vi "HOL_Trajectory_SampleReverseTEST_CONSTORIENT.vi"(9 "Time":dbl, 11 "InputTRAJECTORY":T5 {"States"."POSE"."ROTATION"."SIN" format="%13.4f"; "States"."POSE"."ROTATION"."COS" format="%13.4f"; "States"."POSE"."ROTATION"."VALUE" format="%13.4f"; "States"."POSE"."TRANSLATION"."Y" format="%14.3f"; "States"."POSE"."TRANSLATION"."X" format="%14.3f"; "TotalTImeSecs" format="%20.3f"}) -> (3 "OutputTRAJ_STATE":T1={"TimeSeconds"=0.0, "Velocity"=0.0, "Acceleration"=0.0, "POSE"={"TRANSLATION"={"X"=0.0, "Y"=0.0}, "ROTATION"={"VALUE"=0.0, "COS"=1.0, "SIN"=0.0}}, "Curvature"=0.0} {"POSE"."ROTATION"."SIN" format="%13.4f"; "POSE"."ROTATION"."COS" format="%13.4f"; "POSE"."ROTATION"."VALUE" format="%13.4f"; "POSE"."TRANSLATION"."Y" format="%14.3f"; "POSE"."TRANSLATION"."X" format="%14.3f"})   [LabVIEW 2019]
doc: "Sample the trajectory at a point in time. The trajectory is sampled in reverse such that the ending time becomes 0 and the beginning time is the maximum time. The selected trajectory state is then transformed to be relative to end of the trajectory.\n\nThis routine does not exist in WPILIB\n \nParameters:\n - InputTrajectory - The Trajectory data structure\n - time - The point in time since the beginning of the trajectory to sample. (seconds)\n\nReturns:\n - OutputTrajState - The state at that point in time."
uses:
  <vilib>/Rock Robotics/WPI/ThirdParty/JAS_Junk/TrajLib/TRAJECTORY.ctl
  <vilib>/Rock Robotics/WPI/ThirdParty/JAS_Junk/TrajLib/TRAJ_STATE.ctl
  <vilib>/Rock Robotics/WPI/ThirdParty/JAS_Junk/TrajLib/POSE2D.ctl
  <vilib>/Rock Robotics/WPI/ThirdParty/JAS_Junk/TrajLib/TRANSLATION2D.ctl
  <vilib>/Rock Robotics/WPI/ThirdParty/JAS_Junk/TrajLib/ROTATION2D.ctl
  <vilib>/Rock Robotics/WPI/ThirdParty/JAS_Junk/TrajLib/Translation_Create.vi
  <vilib>/Rock Robotics/WPI/ThirdParty/JAS_Junk/TrajLib/Trajectory_Library.lvlib
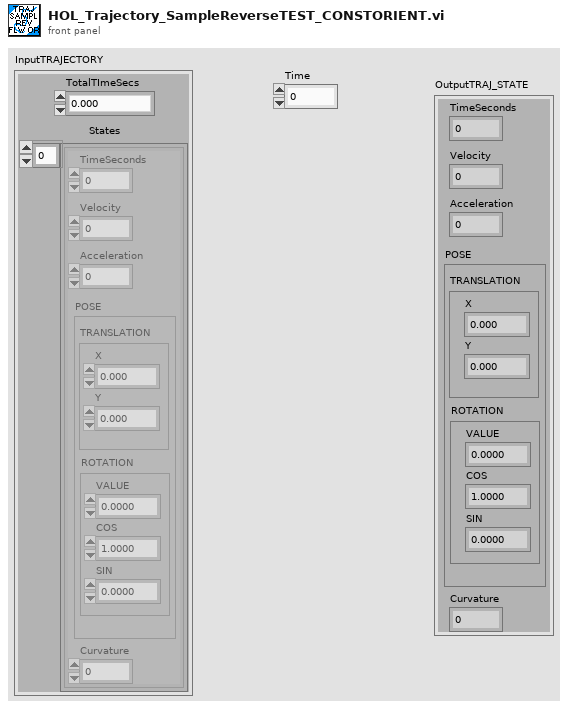
[diagram p1: front panel]
types:
  T1 = typedef "Trajectory_Library.lvlib/TRAJ_STATE.ctl" = cluster{"TimeSeconds":dbl, "Velocity":dbl, "Acceleration":dbl, "POSE":T2, "Curvature":dbl}
  T2 = typedef "Trajectory_Library.lvlib/POSE2D.ctl" = cluster{"TRANSLATION":T3, "ROTATION":T4}
  T3 = typedef "Trajectory_Library.lvlib/TRANSLATION2D.ctl" = cluster{"X":dbl, "Y":dbl}
  T4 = typedef "Trajectory_Library.lvlib/ROTATION2D.ctl" = cluster{"VALUE":dbl, "COS":dbl, "SIN":dbl}
  T5 = typedef "Trajectory_Library.lvlib/TRAJECTORY.ctl" = cluster{"TotalTImeSecs":dbl, "States":T1[]}
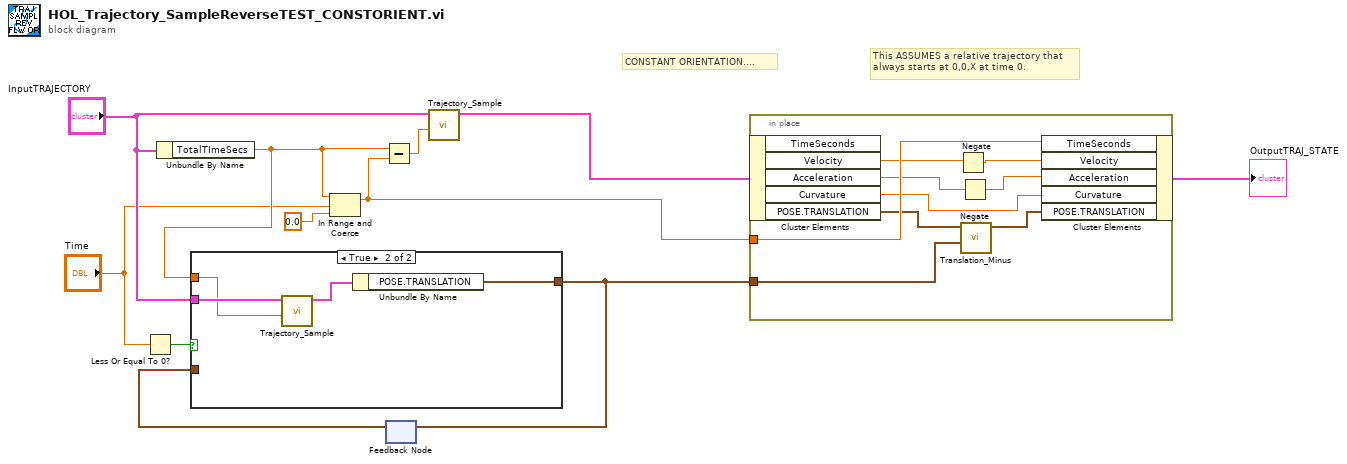
[diagram p0: block diagram]
diagram:
  # "This ASSUMES a relative trajectory that \nalways starts at 0,0,X at time 0."
  # "CONSTANT ORIENTATION...."
  n1 = Less Or Equal To 0?(x="Time") -> (x <= 0?=w11:bool)
  n2 = Unbundle By Name("InputTRAJECTORY") -> ("TotalTImeSecs"=w4:dbl)
  n3 = In Range and Coerce(upper limit=w4, x="Time", lower limit=0.0) -> (coerced(x)=w2:dbl)  [unwired: 1 out]
  n4 = Subtract(x=w4, y=w2) -> (x-y=w1:dbl)
  n5 = feedback #1() -> (w7:T3)  [unwired: 1 in]
  n6 = case shown="True" w11 {
    tunnel: "InputTRAJECTORY" -> [_ w15]
    tunnel: w4 -> [_ w14]
    tunnel: [w12 w13] -> w6
    tunnel: w7 -> [w12 _]
    frame False {
    }
    frame True {
      n7 = call <vilib>:"Trajectory_Sample.vi"("Time"=w14, "InputTRAJECTORY"=w15) -> ("OutputTRAJ_STATE"=w16:T1)  [unwired: 9 in]
      n8 = Unbundle By Name(w16) -> ("POSE.TRANSLATION"=w13:T3)
    }
  }
  n9 = feedback-in #1(w6) -> ()
  n10 = call <vilib>:"Trajectory_Sample.vi"("Time"=w1, "InputTRAJECTORY"="InputTRAJECTORY") -> ("OutputTRAJ_STATE"=w9:T1)  [unwired: 9 in]
  n11 = in-place {
    in-place-border: w2 -> [w24]
    in-place-border: w6 -> [w17]
    n12 = in-place-cluster #2(w9) -> ("Velocity"=w23:dbl, "Acceleration"=w21:dbl, "Curvature"=w20:dbl, "POSE.TRANSLATION"=w19:T3)  [unwired: 1 out]
    n13 = Negate(x=w23) -> (-x=w22:dbl)
    n14 = Negate(x=w21) -> ()  [unwired: 1 out]
    n15 = call <vilib>:"Translation_Minus.vi"("other Translation"=w17, "In Translation"=w19) -> ("Out Translation"=w18:T3)  [unwired: 9 in]
    n16 = in-place-cluster #2("TimeSeconds"=w24, "Velocity"=w22, "Acceleration"=w21, "Curvature"=w20, "POSE.TRANSLATION"=w18) -> (→"OutputTRAJ_STATE":T1)
  }
